vi "Pre Launch Init.vi"(11 "TestStand Controller in":refnum<class "Controller API.lvclass">) -> (0 "error out":errorcluster, 3 "TestStand Controller out":refnum<class "Controller API.lvclass">)   [LabVIEW 2017, in "Controller API.lvlib" / "Controller API.lvclass"]
doc: "(<B>Filename</B>: Actor Framework.lvlib:Actor.lvclass:Pre Launch Init.vi)\n\nDefines behavior that occurs after the Launch Actor method is invoked but before the actor's Actor Core method begins running.\n\nThe Pre Launch Init method is guaranteed to finish before the Launch Actor method returns to its caller and before the actor itself receives any messages. Any references that the Pre Launch Init method obtains are guaranteed to have the same lifetime as the actor itself. Any errors that the Pre Launch Init method returns will abort the launch.\n\nBy default, this method does nothing. A descendant class may override it to define behavior."
uses:
  Controller API.lvclass
  C:/Program Files (x86)/National Instruments/LabVIEW 2017/vi.lib/ActorFramework/Actor/Actor.lvclass
  <vilib>/ActorFramework/Actor/Actor.lvclass/Actor.ctl
  <vilib>/ActorFramework/Message Enqueuer/Message Enqueuer.lvclass/Message Enqueuer.ctl
  <vilib>/ActorFramework/Message Enqueuer/Init from Existing Queue.vi
  <vilib>/ActorFramework/Message Enqueuer/Enqueue.vi
  MAL-Framework/user.lib/Common Components/Controller/Messages/Measurements Scan Msg/Measurements Scan Msg.lvclass
  C:/Program Files (x86)/National Instruments/LabVIEW 2017/vi.lib/ActorFramework/Message/Message.lvclass
  <vilib>/ActorFramework/Message Priority Queue/Priority Enqueue.vi
  MAL-Framework/user.lib/Common Components/Controller/Controller.lvclass
  <vilib>/ActorFramework/Message Enqueuer/Message Enqueuer.lvclass
  <vilib>/ActorFramework/Actor/Actor.lvclass
  MAL-Framework/user.lib/Common Components/Controller/Messages/Scan Hardware Message/Scan Hardware Message.lvclass
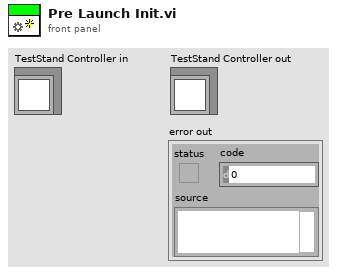
[diagram p1: front panel]
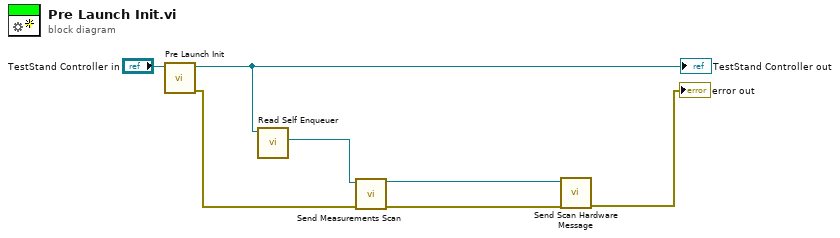
[diagram p0: block diagram]
diagram:
  n1 = call-parent "Pre Launch Init.vi"("Controller in"="TestStand Controller in") -> ("error out"=w2:errorcluster, "Controller out"=w6:refnum<class "Controller API.lvclass">)  [unwired: 9 in]
  "TestStand Controller out" <- w6
  n2 = call <vilib>:"Read Self Enqueuer.vi"("Actor"=w6) -> ("Self Enqueuer"=w5:refnum<class "Message Enqueuer.lvclass">)  [unwired: 10 in]
  n3 = call "Send Measurements Scan.vi"("error in (no error)"=w2, "Message Enqueuer"=w5) -> ("error out"=w3:errorcluster, "Message Enqueuer out"=w4:refnum<class "Message Enqueuer.lvclass">)  [unwired: 8 in]
  n4 = call "Send Scan Hardware Message.vi"("error in (no error)"=w3, "Message Enqueuer in"=w4) -> ("error out"=→"error out":errorcluster)  [unwired: 8 in, 1 out]
